vi "ReadBankChannelNode.vi"(8 "Error In":errorcluster, 11 "Bank Channel Node In":refnum<k20>) -> (0 "Error Out":errorcluster, 2 "Name":string, 3 "Bank Channel Node Out":refnum<k20>)   [LabVIEW 2012]
uses:
  <vilib>/xml/NI_XML.lvlib
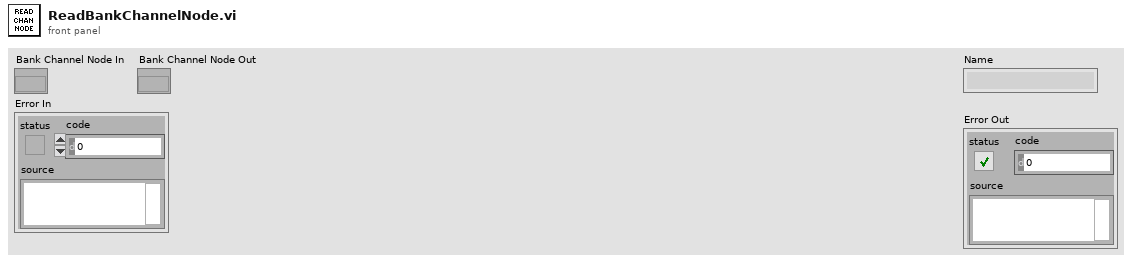
[diagram p1: front panel]
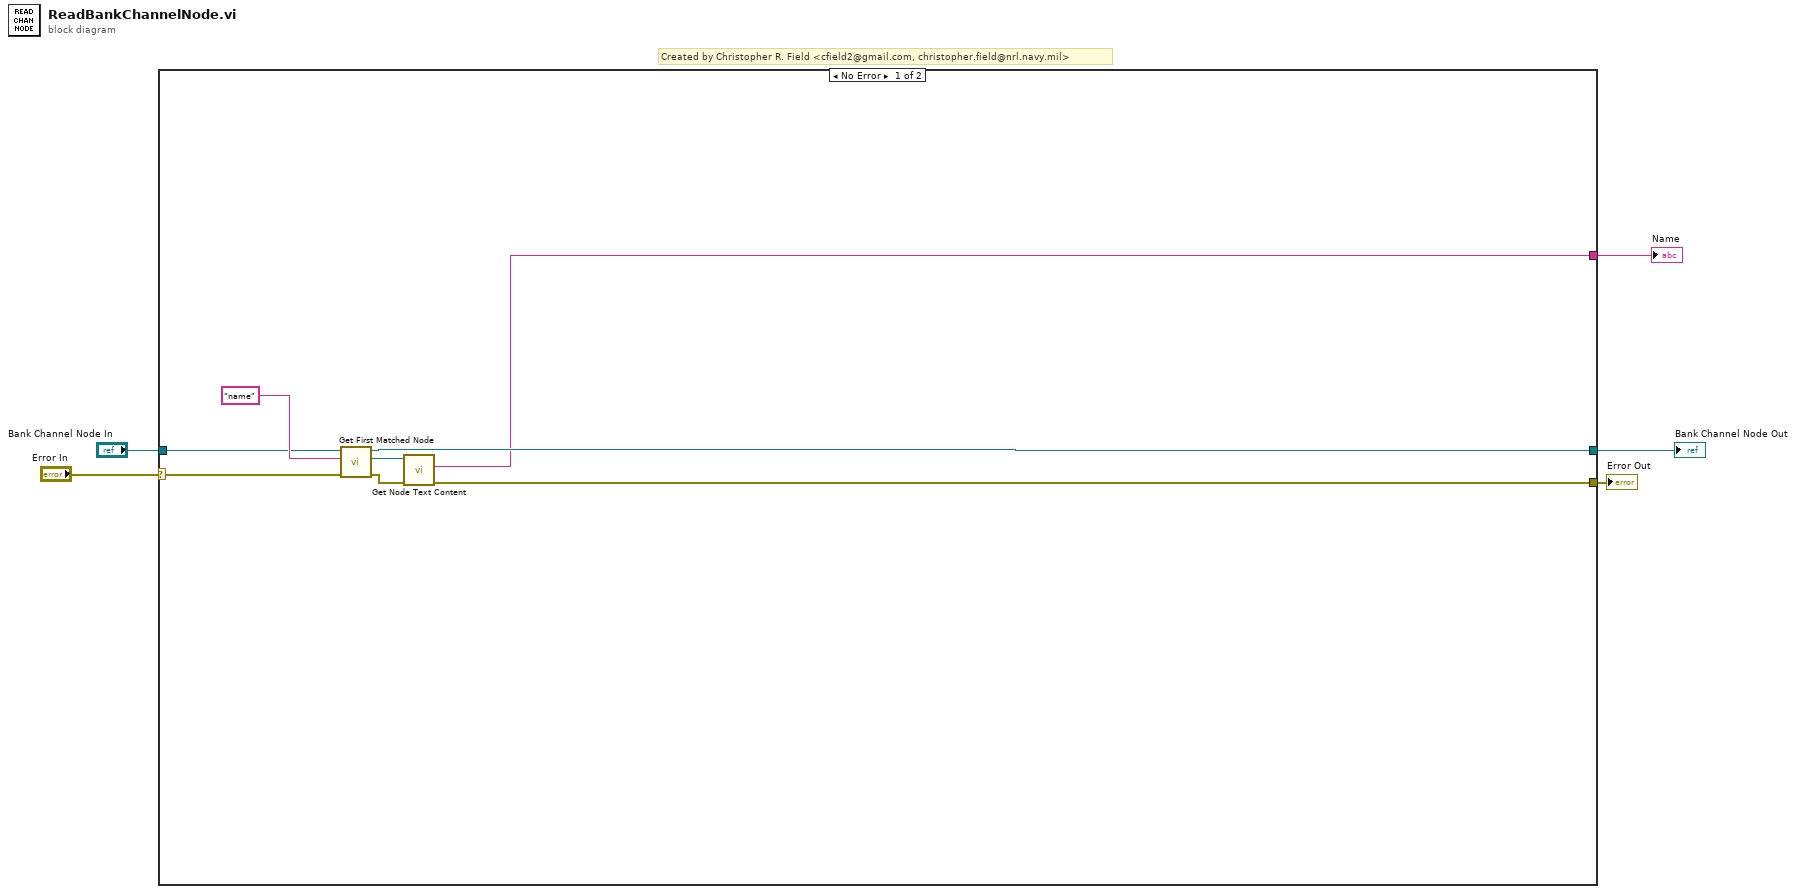
[diagram p0: block diagram]
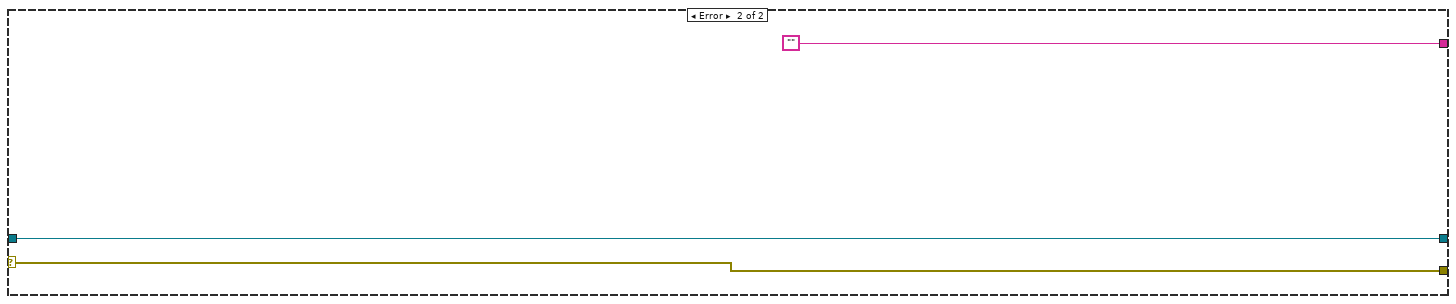
[diagram p2: hidden frame]
diagram:
  # "Created by Christopher R. Field <cfield2@gmail.com, christopher.field@nrl.navy.mil>"
  n1 = case shown="No Error" "Error In" {
    selector: "Error In" -> [w11 w15]
    tunnel: "Bank Channel Node In" -> [w12 w16]
    tunnel: [w8 w15] -> w3
    tunnel: [w7 w16] -> w2
    tunnel: [w6 ""] -> w1
    frame No Error {
      n2 = call <vilib>:"Get First Matched Node.vi"("error in (no error)"=w11, "XPath expression"="name", "node in"=w12) -> ("error out"=w9:errorcluster, "node result"=w10:refnum<k20>, "node out"=w7:refnum<k20>)  [unwired: 6 in]
      n3 = call <vilib>:"Get Node Text Content.vi"("error in (no error)"=w9, "node in"=w10) -> ("error out"=w8:errorcluster, "node text"=w6:string)  [unwired: 7 in, 1 out]
    }
    frame Error {
    }
  }
  "Error Out" <- w3
  "Bank Channel Node Out" <- w2
  "Name" <- w1
